vi "HandleObservationSync_002.vi"(8 "error in (no error)":errorcluster, 11 "S4GUI in":refnum<class "S4GUI.lvclass">) -> (0 "error out":errorcluster, 3 "S4GUI out":refnum<class "S4GUI.lvclass">)   [LabVIEW 2018, in "S4GUI.lvclass"] (continued)
            tunnel: ["" ("Error Msg") "ERROR: Lost channel 1 connection... - HandleObservationSync.vi state 308" ("Error Msg") "ERROR: Lost channel 2 connection...- HandleObservationSync.vi state 308" ("Error Msg") "ERROR: Lost channels 1 and 2 connection...- HandleObservationSync.vi state 308" ("Error Msg") "ERROR: Lost channel 3 connection...- HandleObservationSync.vi state 308" ("Error Msg") "ERROR: Lost channels 1 and  3 connection...- HandleObservationSync.vi state 308" ("Error Msg") "ERROR:  Lost channels 2 and  3 connection...- HandleObservationSync.vi state 308" ("Error Msg") "ERROR:  Lost channels 1, 2 and  3 connection...- HandleObservationSync.vi state 308" ("Error Msg") "ERROR: Lost channel 4 connection...- HandleObservationSync.vi state 308" ("Error Msg") "ERROR:  Lost channels 1 and 4 connection...- HandleObservationSync.vi state 308" ("Error Msg") "ERROR:  Lost channels 2 and 4 connection...- HandleObservationSync.vi state 308" ("Error Msg") "ERROR: Lost channels 1, 2 and 4 connection...- HandleObservationSync.vi state 308" ("Error Msg") "ERROR: Lost channels 3 and 4 connection...- HandleObservationSync.vi state 308" ("Error Msg") "ERROR: Lost channels 1, 3 and 4 connection...- HandleObservationSync.vi state 308" ("Error Msg") "ERROR: Lost channels 2, 3 and 4 connection...- HandleObservationSync.vi state 308" ("Error Msg") "ERROR: Lost channels 1, 2, 3 and 4 connection...- HandleObservationSync.vi state 308" ("Error Msg")] -> w2599
            frame 0, Default {
              n1014 = Tick Count (ms)() -> (millisecond timer value=w2631:u32)
              n1015 = Increment(x=w2634) -> (x+1=w2633:u32)
              n1016 = local write "time1"(w2631) -> ()
            }
            frame 1 {
            }
            frame 2 {
            }
            frame 3 {
            }
            frame 4 {
            }
            frame 5 {
            }
            frame 6 {
            }
            frame 7 {
            }
            frame 8 {
            }
            frame 9 {
            }
            frame 10 {
            }
            frame 11 {
            }
            frame 12 {
            }
            frame 13 {
            }
            frame 14 {
            }
            frame 15 {
            }
          }
          n1017 = Bundle By Name(cluster=w2608, "Obs_state"=w2598, "Error Msg"=w2599) -> (w2625:refnum<class "S4GUI.lvclass">)
        }
        frame 309 {
          # "Se wait_expose=T, não envia\no EXPOSE do estado 310\n(1o EXPOSE já foi enviado).\n\nNeste caso, vai para:\n* 310 se houver mais \n   de 1 posição da lamina ou para \n* 327 se houver apenas 1 posição\n   da lâmina"
          # "T: mode EXPOSE\nF: mode FIRE"
          # "Espera todos os canais chegarem ao estado ACTIVE\n(estados 54 e 55 de Channel:Run.vi)\n   OU\nTodos os canais incrementarem o Seqs_done. (OV 20240821)"
          n1018 = Unbundle By Name(w2754) -> ("seqAtual"=w2753:u32)
          n1019 = call-dynamic "Read AcquisitionA.vi"("error in (no error)"=w2816, "S4ACS_GUI in"=w2754) -> ("error out"=w2796:errorcluster, "Acquisition.lvclass"=w2797:refnum<class "Acquisition.lvclass">, "S4ACS_GUI out"=w2818:refnum<class "S4GUI.lvclass">)  [unwired: 7 in]
          n1020 = call "Read connection.vi"("error in (no error)"=w2796, "Server in"=w2797) -> ("error out"=w2798:errorcluster, "connection"=w2800:bool, "Server out"=w2799:refnum<class "Acquisition.lvclass">)  [unwired: 7 in]
          n1021 = case shown="True" w2800 {
            tunnel: [w2953 w2977] -> w2819
            tunnel: [w2952 w2976] -> w2817
            tunnel: w2799 -> [w2953 w2969]
            tunnel: w2798 -> [w2952 w2968]
            tunnel: [TRUE w2967] -> w2779
            tunnel: [FALSE w2961] -> w2775
            tunnel: [TRUE w2955] -> w2758
            tunnel: w2753 -> [_ w2954]
            frame False {
            }
            frame True {
              n1022 = call-dynamic "Read Channel.vi"("error in (no error)"=w2968, "Acquisition in"=w2969) -> ("error out"=w2958:errorcluster, "Channel.lvclass"=w2960:refnum<class "Channel.lvclass">, "Acquisition out"=w2978:refnum<class "Acquisition.lvclass">)  [unwired: 7 in]
              n1023 = call-dynamic "Read SequesDone.vi"("error in (no error)"=w2958, "Channel in"=w2960) -> ("error out"=w2957:errorcluster, "SequesDoneRaw"=w2956:u32, "Channel out"=w2959:refnum<class "Channel.lvclass">)  [unwired: 6 in, 1 out]
              n1024 = Equal?(x=w2956, y=w2954) -> (x = y?=w2955:bool)
              n1025 = call-dynamic "Read wait_expose.vi"("error in (no error)"=w2957, "Channel in"=w2959) -> ("error out"=w2962:errorcluster, "wait_expose"=w2961:bool, "Channel out"=w2963:refnum<class "Channel.lvclass">)  [unwired: 7 in]
              n1026 = call-dynamic "Read State Machine.vi"("error in (no error)"=w2962, "Device in"=w2963) -> ("error out"=w2970:errorcluster, "State Machine.lvclass"=w2972:refnum<class "State Machine.lvclass">, "Device out"=w2974:refnum<class "Channel.lvclass">)  [unwired: 7 in]
              n1027 = call-dynamic "Read State.vi"("error in (no error)"=w2970, "State Machine in"=w2972) -> ("error out"=w2964:errorcluster, "State"=w2966:i32, "State Machine out"=w2971:refnum<class "State Machine.lvclass">)  [unwired: 7 in]
              n1028 = Greater?(x=w2966, y=53) -> (0:w2967:bool)
              n1029 = call-dynamic "Write State Machine.vi"("error in (no error)"=w2964, "State Machine.lvclass"=w2971, "Device in"=w2974) -> ("error out"=w2973:errorcluster, "Device out"=w2975:refnum<class "Channel.lvclass">)  [unwired: 7 in]
              n1030 = call-dynamic "Write Channel.vi"("error in (no error)"=w2973, "Channel.lvclass"=w2975, "Acquisition in"=w2978) -> ("error out"=w2976:errorcluster, "Acquisition out"=w2977:refnum<class "Acquisition.lvclass">)  [unwired: 7 in]
            }
          }
          n1031 = call-dynamic "Write AcquisitionA.vi"("error in (no error)"=w2817, "Acquisition.lvclass"=w2819, "S4ACS_GUI in"=w2818) -> ("error out"=w2813:errorcluster, "S4ACS_GUI out"=w2814:refnum<class "S4GUI.lvclass">)  [unwired: 7 in]
          n1032 = call "Read AcquisitionB.vi"("error in (no error)"=w2813, "S4ACS_GUI in"=w2814) -> ("error out"=w2793:errorcluster, "Acquisition.lvclass"=w2795:refnum<class "Acquisition.lvclass">, "S4ACS_GUI out"=w2811:refnum<class "S4GUI.lvclass">)  [unwired: 7 in]
          n1033 = call "Read connection.vi"("error in (no error)"=w2793, "Server in"=w2795) -> ("error out"=w2792:errorcluster, "connection"=w2791:bool, "Server out"=w2794:refnum<class "Acquisition.lvclass">)  [unwired: 7 in]
          n1034 = case shown="True" w2791 {
            tunnel: w2794 -> [w2923 w2948]
            tunnel: w2792 -> [w2922 w2947]
            tunnel: [w2923 w2945] -> w2812
            tunnel: [w2922 w2944] -> w2810
            tunnel: [TRUE w2935] -> w2778
            tunnel: [FALSE ("expose") w2931] -> w2774
            tunnel: [TRUE w2925] -> w2760
            tunnel: w2753 -> [_ w2924]
            frame False {
            }
            frame True {
              n1035 = call-dynamic "Read Channel.vi"("error in (no error)"=w2947, "Acquisition in"=w2948) -> ("error out"=w2927:errorcluster, "Channel.lvclass"=w2930:refnum<class "Channel.lvclass">, "Acquisition out"=w2946:refnum<class "Acquisition.lvclass">)  [unwired: 7 in]
              n1036 = call-dynamic "Read SequesDone.vi"("error in (no error)"=w2927, "Channel in"=w2930) -> ("error out"=w2926:errorcluster, "SequesDoneRaw"=w2928:u32, "Channel out"=w2929:refnum<class "Channel.lvclass">)  [unwired: 6 in, 1 out]
              n1037 = Equal?(x=w2928, y=w2924) -> (x = y?=w2925:bool)
              n1038 = call-dynamic "Read wait_expose.vi"("error in (no error)"=w2926, "Channel in"=w2929) -> ("error out"=w2932:errorcluster, "wait_expose"=w2931:bool, "Channel out"=w2933:refnum<class "Channel.lvclass">)  [unwired: 7 in]
              n1039 = call-dynamic "Read State Machine.vi"("error in (no error)"=w2932, "Device in"=w2933) -> ("error out"=w2938:errorcluster, "State Machine.lvclass"=w2940:refnum<class "State Machine.lvclass">, "Device out"=w2942:refnum<class "Channel.lvclass">)  [unwired: 7 in]
              n1040 = call-dynamic "Read State.vi"("error in (no error)"=w2938, "State Machine in"=w2940) -> ("error out"=w2937:errorcluster, "State"=w2934:i32, "State Machine out"=w2939:refnum<class "State Machine.lvclass">)  [unwired: 7 in]
              n1041 = Greater?(x=w2934, y=53) -> (0:w2935:bool)
              n1042 = call-dynamic "Write State Machine.vi"("error in (no error)"=w2937, "State Machine.lvclass"=w2939, "Device in"=w2942) -> ("error out"=w2941:errorcluster, "Device out"=w2943:refnum<class "Channel.lvclass">)  [unwired: 7 in]
              n1043 = call-dynamic "Write Channel.vi"("error in (no error)"=w2941, "Channel.lvclass"=w2943, "Acquisition in"=w2946) -> ("error out"=w2944:errorcluster, "Acquisition out"=w2945:refnum<class "Acquisition.lvclass">)  [unwired: 7 in]
            }
          }
          n1044 = call "Write AcquisitionB.vi"("error in (no error)"=w2810, "Acquisition.lvclass"=w2812, "S4ACS_GUI in"=w2811) -> ("error out"=w2806:errorcluster, "S4ACS_GUI out"=w2805:refnum<class "S4GUI.lvclass">)  [unwired: 7 in]
          n1045 = call-dynamic "Read AcquisitionC.vi"("error in (no error)"=w2806, "S4ACS_GUI in"=w2805) -> ("error out"=w2788:errorcluster, "Acquisition.lvclass"=w2790:refnum<class "Acquisition.lvclass">, "S4ACS_GUI out"=w2808:refnum<class "S4GUI.lvclass">)  [unwired: 7 in]
          n1046 = call "Read connection.vi"("error in (no error)"=w2788, "Server in"=w2790) -> ("error out"=w2787:errorcluster, "connection"=w2786:bool, "Server out"=w2789:refnum<class "Acquisition.lvclass">)  [unwired: 7 in]
          n1047 = case shown="True" w2786 {
            tunnel: [w2892 w2913] -> w2809
            tunnel: [w2893 w2912] -> w2807
            tunnel: w2789 -> [w2893 w2908]
            tunnel: w2787 -> [w2892 w2907]
            tunnel: [TRUE w2904] -> w2777
            tunnel: [FALSE ("expose") w2901] -> w2773
            tunnel: [TRUE w2895] -> w2759
            tunnel: w2753 -> [_ w2894]
            frame False {
            }
            frame True {
              n1048 = call-dynamic "Read Channel.vi"("error in (no error)"=w2907, "Acquisition in"=w2908) -> ("error out"=w2900:errorcluster, "Channel.lvclass"=w2899:refnum<class "Channel.lvclass">, "Acquisition out"=w2911:refnum<class "Acquisition.lvclass">)  [unwired: 7 in]
              n1049 = call-dynamic "Read SequesDone.vi"("error in (no error)"=w2900, "Channel in"=w2899) -> ("error out"=w2896:errorcluster, "SequesDoneRaw"=w2897:u32, "Channel out"=w2898:refnum<class "Channel.lvclass">)  [unwired: 6 in, 1 out]
              n1050 = Equal?(x=w2897, y=w2894) -> (x = y?=w2895:bool)
              n1051 = call-dynamic "Read wait_expose.vi"("error in (no error)"=w2896, "Channel in"=w2898) -> ("error out"=w2902:errorcluster, "wait_expose"=w2901:bool, "Channel out"=w2903:refnum<class "Channel.lvclass">)  [unwired: 7 in]
              n1052 = call-dynamic "Read State Machine.vi"("error in (no error)"=w2902, "Device in"=w2903) -> ("error out"=w2909:errorcluster, "State Machine.lvclass"=w2917:refnum<class "State Machine.lvclass">, "Device out"=w2915:refnum<class "Channel.lvclass">)  [unwired: 7 in]
              n1053 = call-dynamic "Read State.vi"("error in (no error)"=w2909, "State Machine in"=w2917) -> ("error out"=w2910:errorcluster, "State"=w2905:i32, "State Machine out"=w2918:refnum<class "State Machine.lvclass">)  [unwired: 7 in]
              n1054 = Greater?(x=w2905, y=53) -> (0:w2904:bool)
              n1055 = call-dynamic "Write State Machine.vi"("error in (no error)"=w2910, "State Machine.lvclass"=w2918, "Device in"=w2915) -> ("error out"=w2916:errorcluster, "Device out"=w2914:refnum<class "Channel.lvclass">)  [unwired: 7 in]
              n1056 = call-dynamic "Write Channel.vi"("error in (no error)"=w2916, "Channel.lvclass"=w2914, "Acquisition in"=w2911) -> ("error out"=w2913:errorcluster, "Acquisition out"=w2912:refnum<class "Acquisition.lvclass">)  [unwired: 7 in]
            }
          }
          n1057 = call-dynamic "Write AcquisitionC.vi"("error in (no error)"=w2809, "Acquisition.lvclass"=w2807, "S4ACS_GUI in"=w2808) -> ("error out"=w2785:errorcluster, "S4ACS_GUI out"=w2801:refnum<class "S4GUI.lvclass">)  [unwired: 7 in]
          n1058 = call-dynamic "Read AcquisitionD.vi"("error in (no error)"=w2785, "S4ACS_GUI in"=w2801) -> ("error out"=w2781:errorcluster, "Acquisition.lvclass"=w2784:refnum<class "Acquisition.lvclass">, "S4ACS_GUI out"=w2803:refnum<class "S4GUI.lvclass">)  [unwired: 7 in]
          n1059 = call "Read connection.vi"("error in (no error)"=w2781, "Server in"=w2784) -> ("error out"=w2782:errorcluster, "connection"=w2780:bool, "Server out"=w2783:refnum<class "Acquisition.lvclass">)  [unwired: 7 in]
          n1060 = case shown="True" w2780 {
            tunnel: [w2863 w2887] -> w2804
            tunnel: [w2862 w2886] -> w2802
            tunnel: [TRUE w2875] -> w2776
            tunnel: w2783 -> [w2863 w2878]
            tunnel: w2782 -> [w2862 w2877]
            tunnel: [FALSE ("expose") w2871] -> w2772
            tunnel: [TRUE w2865] -> w2761
            tunnel: w2753 -> [_ w2864]
            frame False {
            }
            frame True {
              n1061 = call-dynamic "Read Channel.vi"("error in (no error)"=w2877, "Acquisition in"=w2878) -> ("error out"=w2869:errorcluster, "Channel.lvclass"=w2870:refnum<class "Channel.lvclass">, "Acquisition out"=w2888:refnum<class "Acquisition.lvclass">)  [unwired: 7 in]
              n1062 = call-dynamic "Read SequesDone.vi"("error in (no error)"=w2869, "Channel in"=w2870) -> ("error out"=w2867:errorcluster, "SequesDoneRaw"=w2868:u32, "Channel out"=w2866:refnum<class "Channel.lvclass">)  [unwired: 6 in, 1 out]
              n1063 = Equal?(x=w2868, y=w2864) -> (x = y?=w2865:bool)
              n1064 = call-dynamic "Read wait_expose.vi"("error in (no error)"=w2867, "Channel in"=w2866) -> ("error out"=w2872:errorcluster, "wait_expose"=w2871:bool, "Channel out"=w2873:refnum<class "Channel.lvclass">)  [unwired: 7 in]
              n1065 = call-dynamic "Read State Machine.vi"("error in (no error)"=w2872, "Device in"=w2873) -> ("error out"=w2880:errorcluster, "State Machine.lvclass"=w2882:refnum<class "State Machine.lvclass">, "Device out"=w2884:refnum<class "Channel.lvclass">)  [unwired: 7 in]
              n1066 = call-dynamic "Read State.vi"("error in (no error)"=w2880, "State Machine in"=w2882) -> ("error out"=w2879:errorcluster, "State"=w2874:i32, "State Machine out"=w2881:refnum<class "State Machine.lvclass">)  [unwired: 7 in]
              n1067 = Greater?(x=w2874, y=53) -> (0:w2875:bool)
              n1068 = call-dynamic "Write State Machine.vi"("error in (no error)"=w2879, "State Machine.lvclass"=w2881, "Device in"=w2884) -> ("error out"=w2883:errorcluster, "Device out"=w2885:refnum<class "Channel.lvclass">)  [unwired: 7 in]
              n1069 = call-dynamic "Write Channel.vi"("error in (no error)"=w2883, "Channel.lvclass"=w2885, "Acquisition in"=w2888) -> ("error out"=w2886:errorcluster, "Acquisition out"=w2887:refnum<class "Acquisition.lvclass">)  [unwired: 7 in]
            }
          }
          n1070 = call-dynamic "Write AcquisitionD.vi"("error in (no error)"=w2802, "Acquisition.lvclass"=w2804, "S4ACS_GUI in"=w2803) -> ("error out"=w2770:errorcluster, "S4ACS_GUI out"=w2771:refnum<class "S4GUI.lvclass">)  [unwired: 7 in]
          n1071 = Compound Arithmetic op=OR(w2775, w2774, w2773, w2772) -> (w2763:bool)
          n1072 = Compound Arithmetic op=AND(w2758, w2760, w2759, w2761) -> (w2756:bool)
          n1073 = Compound Arithmetic op=AND(w2779, w2778, w2777, w2776) -> (w2757:bool)
          n1074 = Or(x=w2757, y=w2756) -> (x .or. y?=w2755:bool)
          n1075 = call-dynamic "VerifWavePlate.vi"("error in (no error)"=w2770, "S4GUI in"=w2771) -> ("error out"=w2767:errorcluster, "One Position"=w2769:bool, "S4GUI out"=w2768:refnum<class "S4GUI.lvclass">)  [unwired: 7 in]
          n1076 = case shown="True" w2769 {
            tunnel: w2768 -> [w2840 w2857]
            tunnel: [u32 312 ("t") u32 327 ("t")] -> w2765
            tunnel: [w2840 w2843] -> w2764
            tunnel: w2767 -> [w2838 w2842]
            tunnel: [w2838 w2841] -> w2766
            frame False {
            }
            frame True {
              # "Recarrega SEQ, antes de desviar\n para tratamento de fotometria."
              n1077 = call "Read Instrument.lvclass.vi"("error in (no error)"=w2842, "S4ACS_GUI in"=w2857) -> ("error out"=w2852:errorcluster, "Instrument.lvclass"=w2856:refnum<class "Instrument.lvclass">, "S4ACS_GUI out"=w2855:refnum<class "S4GUI.lvclass">)  [unwired: 7 in]
              n1078 = call "Read WPROT.vi"("error in (no error)"=w2852, "Instrument in"=w2856) -> ("error out"=w2845:errorcluster, "Opt_Selector.lvclass"=w2848:refnum<class "Opt_Selector.lvclass">, "Instrument out"=w2853:refnum<class "Instrument.lvclass">)  [unwired: 7 in]
              n1079 = call-dynamic "Read sequencia_ant.vi"("error in (no error)"=w2845, "Opt_Selector in"=w2848) -> ("error out"=w2850:errorcluster, "sequencia_ant"=w2849:u16, "Opt_Selector out"=w2847:refnum<class "Opt_Selector.lvclass">)  [unwired: 7 in]
              n1080 = call-dynamic "Write sequencia.vi"("error in (no error)"=w2850, "sequencia"=w2849, "Opt_Selector in"=w2847) -> ("error out"=w2844:errorcluster, "Opt_Selector out"=w2846:refnum<class "Opt_Selector.lvclass">)  [unwired: 7 in]
              n1081 = call "Write WPROT.vi"("error in (no error)"=w2844, "Opt_Selector.lvclass"=w2846, "Instrument in"=w2853) -> ("error out"=w2851:errorcluster, "Instrument out"=w2854:refnum<class "Instrument.lvclass">)  [unwired: 7 in]
              n1082 = call "Write Instrument.lvclass.vi"("error in (no error)"=w2851, "Instrument.lvclass"=w2854, "S4ACS_GUI in"=w2855) -> ("error out"=w2841:errorcluster, "S4ACS_GUI out"=w2843:refnum<class "S4GUI.lvclass">)  [unwired: 7 in]
            }
          }
          n1083 = case shown="True" w2755 {
            tunnel: w2764 -> [w2821 w2837]
            tunnel: [w2827 w2836] -> w2762
            tunnel: w2765 -> [_ w2834]
            frame False {
              # "Aguardando iniciar exposição por 5s"
              n1084 = Tick Count (ms)() -> (millisecond timer value=w2826:u32)
              n1085 = local read "time1"() -> (w2820:u32)
              n1086 = Subtract(x=w2826, y=w2820) -> (x-y=w2823:u32)
              n1087 = To Double Precision Float(number=w2823) -> (double precision float=w2825:dbl)
              n1088 = Less?(x=5000.0 ("y"), y=w2825) -> (x < y?=w2824:bool)
              n1089 = case shown="True" w2824 {
                tunnel: w2821 -> [w2828 w2832]
                tunnel: [w2828 w2831] -> w2827
                frame False {
                }
                frame True {
                  n1090 = Bundle By Name(cluster=w2832, "Obs_state"=u32 1, "Error Msg"="ERROR: Acquisition Timeout. HandleObservationSync.vi - state 309.") -> (w2831:refnum<class "S4GUI.lvclass">)
                }
              }
            }
            frame True {
              # "Iniciou aquisição..."
              n1091 = Tick Count (ms)() -> (millisecond timer value=→"time308":u32)
              n1092 = Tick Count (ms)() -> (millisecond timer value=w2835:u32)
              n1093 = Bundle By Name(cluster=w2837, "Obs_state"=w2834) -> (w2836:refnum<class "S4GUI.lvclass">)
              n1094 = local write "time307"(w2835) -> ()
              n1095 = local write "time1"(w2835) -> ()
            }
          }
          n1096 = Bundle By Name(cluster=w2762, "mode EXPOSE"=w2763) -> (w2815:refnum<class "S4GUI.lvclass">)
        }
        frame 312 {
          # "Verifcando avanço de SEQUENCIA:"
          # "T=canais receberam STOP"
          # "T= Todos os canais ativos na mesma sequencia;\nF= Canais com sequencia diferente"
          # "Todos os SEQ_DONE \nsão iguais a SeqAtual?\nSe sim, avança lâmina."
          # "Exemplo:\nSET #CYCLES 3\nSET #SEQ 4\ntotal de sequencias: 3 x 4 = 12\n\nseq.        CYCLES_DONE           SEQS_DONE\n1a.                     0                                 0\n2a.                     0                                 1 \n3a.                     0                                 2 \n4a.                     0                                 3 \n                          1                                 4\n5a.                     1                                 0 \n6a.                     1                                 1 \n7a.                     1                                 2 \n8a.                     1                                 3 \n                          2                                 4\n9a.                     2                                 0 \n10a.                   2                                 1 \n11a.                   2                                 2 \n12a.                   2                                 3 \n\nfim                    3                                 4"
          n1097 = Unbundle By Name(w3004) -> ("seqAtual"=w3001:u32)
          n1098 = call-dynamic "Read AcquisitionA.vi"("error in (no error)"=w3038, "S4ACS_GUI in"=w3004) -> ("error out"=w3019:errorcluster, "Acquisition.lvclass"=w3020:refnum<class "Acquisition.lvclass">, "S4ACS_GUI out"=w3040:refnum<class "S4GUI.lvclass">)  [unwired: 7 in]
          n1099 = call-dynamic "Read enabled.vi"("error in (no error)"=w3019, "Server in"=w3020) -> ("error out"=w3018:errorcluster, "enabled"=w2993:bool, "Server out"=w3017:refnum<class "Acquisition.lvclass">)  [unwired: 7 in]
          n1100 = case shown="True" w2993 {
            tunnel: w3018 -> [w3189 w3205]
            tunnel: [w3190 w3203] -> w3041
            tunnel: [w3189 w3202] -> w3039
            tunnel: [u32 0 ("SequesDone") w3191] -> w2998
            tunnel: w3017 -> [w3190 w3201]
            tunnel: w3001 -> [_ w3200]
            tunnel: [TRUE w3199] -> w3003
            tunnel: [FALSE ("stopping") w3192] -> w2986
            frame False {
            }
            frame True {
              # "SEQS_DONE = 0,1,2,...,n,0,1,..."
              n1101 = call-dynamic "Read Channel.vi"("error in (no error)"=w3205, "Acquisition in"=w3201) -> ("error out"=w3197:errorcluster, "Channel.lvclass"=w3198:refnum<class "Channel.lvclass">, "Acquisition out"=w3204:refnum<class "Acquisition.lvclass">)  [unwired: 7 in]
              n1102 = call-dynamic "Read SequesDone.vi"("error in (no error)"=w3197, "Channel in"=w3198) -> ("error out"=w3195:errorcluster, "SequesDoneRaw"=w3191:u32, "Channel out"=w3196:refnum<class "Channel.lvclass">)  [unwired: 6 in, 1 out]
              n1103 = Equal?(x=w3191, y=w3200) -> (x = y?=w3199:bool)
              n1104 = call-dynamic "Read stopping.vi"("error in (no error)"=w3195, "Channel in"=w3196) -> ("error out"=w3194:errorcluster, "stopping"=w3192:bool, "Channel out"=w3193:refnum<class "Channel.lvclass">)  [unwired: 7 in]
              n1105 = call-dynamic "Write Channel.vi"("error in (no error)"=w3194, "Channel.lvclass"=w3193, "Acquisition in"=w3204) -> ("error out"=w3202:errorcluster, "Acquisition out"=w3203:refnum<class "Acquisition.lvclass">)  [unwired: 7 in]
            }
          }
          n1106 = call-dynamic "Write AcquisitionA.vi"("error in (no error)"=w3039, "Acquisition.lvclass"=w3041, "S4ACS_GUI in"=w3040) -> ("error out"=w3036:errorcluster, "S4ACS_GUI out"=w3035:refnum<class "S4GUI.lvclass">)  [unwired: 7 in]
          n1107 = call "Read AcquisitionB.vi"("error in (no error)"=w3036, "S4ACS_GUI in"=w3035) -> ("error out"=w3013:errorcluster, "Acquisition.lvclass"=w3016:refnum<class "Acquisition.lvclass">, "S4ACS_GUI out"=w3037:refnum<class "S4GUI.lvclass">)  [unwired: 7 in]
          n1108 = call-dynamic "Read enabled.vi"("error in (no error)"=w3013, "Server in"=w3016) -> ("error out"=w3014:errorcluster, "enabled"=w2992:bool, "Server out"=w3015:refnum<class "Acquisition.lvclass">)  [unwired: 7 in]
          n1109 = case shown="True" w2992 {
            tunnel: w3014 -> [w3169 w3185]
            tunnel: w3015 -> [w3170 w3184]
            tunnel: [u32 0 ("SequesDone") w3171] -> w2995
            tunnel: [w3169 w3183] -> w3034
            tunnel: [w3170 w3182] -> w3033
            tunnel: w3001 -> [_ w3179]
            tunnel: [TRUE w3178] -> w3002
            tunnel: [FALSE ("stopping") w3172] -> w2985
            frame False {
            }
            frame True {
              n1110 = call-dynamic "Read Channel.vi"("error in (no error)"=w3185, "Acquisition in"=w3184) -> ("error out"=w3176:errorcluster, "Channel.lvclass"=w3177:refnum<class "Channel.lvclass">, "Acquisition out"=w3180:refnum<class "Acquisition.lvclass">)  [unwired: 7 in]
              n1111 = call-dynamic "Read SequesDone.vi"("error in (no error)"=w3176, "Channel in"=w3177) -> ("error out"=w3174:errorcluster, "SequesDoneRaw"=w3171:u32, "Channel out"=w3181:refnum<class "Channel.lvclass">)  [unwired: 6 in, 1 out]
              n1112 = Equal?(x=w3171, y=w3179) -> (x = y?=w3178:bool)
              n1113 = call-dynamic "Read stopping.vi"("error in (no error)"=w3174, "Channel in"=w3181) -> ("error out"=w3173:errorcluster, "stopping"=w3172:bool, "Channel out"=w3175:refnum<class "Channel.lvclass">)  [unwired: 7 in]
              n1114 = call-dynamic "Write Channel.vi"("error in (no error)"=w3173, "Channel.lvclass"=w3175, "Acquisition in"=w3180) -> ("error out"=w3183:errorcluster, "Acquisition out"=w3182:refnum<class "Acquisition.lvclass">)  [unwired: 7 in]
            }
          }
          n1115 = call "Write AcquisitionB.vi"("error in (no error)"=w3034, "Acquisition.lvclass"=w3033, "S4ACS_GUI in"=w3037) -> ("error out"=w3026:errorcluster, "S4ACS_GUI out"=w3025:refnum<class "S4GUI.lvclass">)  [unwired: 7 in]
          n1116 = call-dynamic "Read AcquisitionC.vi"("error in (no error)"=w3026, "S4ACS_GUI in"=w3025) -> ("error out"=w3010:errorcluster, "Acquisition.lvclass"=w3012:refnum<class "Acquisition.lvclass">, "S4ACS_GUI out"=w3028:refnum<class "S4GUI.lvclass">)  [unwired: 7 in]
          n1117 = call-dynamic "Read enabled.vi"("error in (no error)"=w3010, "Server in"=w3012) -> ("error out"=w3009:errorcluster, "enabled"=w2991:bool, "Server out"=w3011:refnum<class "Acquisition.lvclass">)  [unwired: 7 in]
          n1118 = case shown="True" w2991 {
            tunnel: [w3149 w3165] -> w3029
            tunnel: [w3150 w3164] -> w3027
            tunnel: w3009 -> [w3149 w3161]
            tunnel: w3011 -> [w3150 w3162]
            tunnel: [u32 0 ("SequesDone") w3151] -> w2994
            tunnel: w3001 -> [_ w3160]
            tunnel: [TRUE w3159] -> w3000
            tunnel: [FALSE ("stopping") w3152] -> w2984
            frame False {
            }
            frame True {
              n1119 = call-dynamic "Read Channel.vi"("error in (no error)"=w3161, "Acquisition in"=w3162) -> ("error out"=w3156:errorcluster, "Channel.lvclass"=w3157:refnum<class "Channel.lvclass">, "Acquisition out"=w3163:refnum<class "Acquisition.lvclass">)  [unwired: 7 in]
              n1120 = call-dynamic "Read SequesDone.vi"("error in (no error)"=w3156, "Channel in"=w3157) -> ("error out"=w3154:errorcluster, "SequesDoneRaw"=w3151:u32, "Channel out"=w3158:refnum<class "Channel.lvclass">)  [unwired: 6 in, 1 out]
              n1121 = Equal?(x=w3151, y=w3160) -> (x = y?=w3159:bool)
              n1122 = call-dynamic "Read stopping.vi"("error in (no error)"=w3154, "Channel in"=w3158) -> ("error out"=w3153:errorcluster, "stopping"=w3152:bool, "Channel out"=w3155:refnum<class "Channel.lvclass">)  [unwired: 7 in]
              n1123 = call-dynamic "Write Channel.vi"("error in (no error)"=w3153, "Channel.lvclass"=w3155, "Acquisition in"=w3163) -> ("error out"=w3165:errorcluster, "Acquisition out"=w3164:refnum<class "Acquisition.lvclass">)  [unwired: 7 in]
            }
          }
          n1124 = call-dynamic "Write AcquisitionC.vi"("error in (no error)"=w3029, "Acquisition.lvclass"=w3027, "S4ACS_GUI in"=w3028) -> ("error out"=w3023:errorcluster, "S4ACS_GUI out"=w3024:refnum<class "S4GUI.lvclass">)  [unwired: 7 in]
          n1125 = call-dynamic "Read AcquisitionD.vi"("error in (no error)"=w3023, "S4ACS_GUI in"=w3024) -> ("error out"=w3006:errorcluster, "Acquisition.lvclass"=w3008:refnum<class "Acquisition.lvclass">, "S4ACS_GUI out"=w3030:refnum<class "S4GUI.lvclass">)  [unwired: 7 in]
          n1126 = call-dynamic "Read enabled.vi"("error in (no error)"=w3006, "Server in"=w3008) -> ("error out"=w3005:errorcluster, "enabled"=w2990:bool, "Server out"=w3007:refnum<class "Acquisition.lvclass">)  [unwired: 7 in]
          n1127 = Build Array(w2993, w2992, w2991, w2990) -> (w2989:bool[])
          n1128 = case shown="True" w2990 {
            tunnel: [w3130 w3145] -> w3032
            tunnel: [w3129 w3144] -> w3031
            tunnel: w3007 -> [w3130 w3143]
            tunnel: w3005 -> [w3129 w3142]
            tunnel: [u32 0 ("SequesDone") w3131] -> w2997
            tunnel: w3001 -> [_ w3140]
            tunnel: [TRUE w3139] -> w2999
            tunnel: [FALSE ("stopping") w3132] -> w2983
            frame False {
            }
            frame True {
              n1129 = call-dynamic "Read Channel.vi"("error in (no error)"=w3142, "Acquisition in"=w3143) -> ("error out"=w3136:errorcluster, "Channel.lvclass"=w3137:refnum<class "Channel.lvclass">, "Acquisition out"=w3141:refnum<class "Acquisition.lvclass">)  [unwired: 7 in]
              n1130 = call-dynamic "Read SequesDone.vi"("error in (no error)"=w3136, "Channel in"=w3137) -> ("error out"=w3134:errorcluster, "SequesDoneRaw"=w3131:u32, "Channel out"=w3138:refnum<class "Channel.lvclass">)  [unwired: 6 in, 1 out]
              n1131 = Equal?(x=w3131, y=w3140) -> (x = y?=w3139:bool)
              n1132 = call-dynamic "Read stopping.vi"("error in (no error)"=w3134, "Channel in"=w3138) -> ("error out"=w3133:errorcluster, "stopping"=w3132:bool, "Channel out"=w3135:refnum<class "Channel.lvclass">)  [unwired: 7 in]
              n1133 = call-dynamic "Write Channel.vi"("error in (no error)"=w3133, "Channel.lvclass"=w3135, "Acquisition in"=w3141) -> ("error out"=w3144:errorcluster, "Acquisition out"=w3145:refnum<class "Acquisition.lvclass">)  [unwired: 7 in]
            }
          }
          n1134 = Boolean Array To Number(Boolean array=w2989) -> (number=w2987:u32)
          n1135 = Compound Arithmetic op=AND(w3003, w3002, w3000, w2999) -> (w2988:bool)
          n1136 = Compound Arithmetic op=OR(w2986, w2985, w2984, w2983) -> (w2982:bool)
          n1137 = case shown="11" w2987 {
            tunnel: w2998 -> [w3049 _ w3061 _ w3070 _ w3076 w3082 _ w3088 w3091 _]
            tunnel: w2997 -> [w3048 w3052 w3057 w3064 w3065 w3073 w3075 _ _ _ _ _]
            tunnel: w2995 -> [w3047 w3050 _ _ w3069 w3071 _ w3081 w3085 _ w3090 _]
            tunnel: w2994 -> [w3046 w3051 w3056 w3062 _ _ _ w3080 w3084 w3087 _ _]
            tunnel: [w3042 w3053 w3058 w3063 w3066 w3072 w3074 w3077 w3083 w3086 w3089 TRUE] -> _
            frame 15 {
              # "A,B,C,D ativos"
              n1138 = Equal?(x=w3049, y=w3047) -> (x = y?=w3045:bool)
              n1139 = Equal?(x=w3046, y=w3048) -> (x = y?=w3043:bool)
              n1140 = Equal?(x=w3047, y=w3046) -> (x = y?=w3044:bool)
              n1141 = Compound Arithmetic op=AND(w3045, w3044, w3043) -> (w3042:bool)
            }
            frame 14 {
              # "B,C e,D ativos"
              n1142 = Equal?(x=w3050, y=w3051) -> (x = y?=w3055:bool)
              n1143 = Equal?(x=w3051, y=w3052) -> (x = y?=w3054:bool)
              n1144 = Compound Arithmetic op=AND(w3055, w3054) -> (w3053:bool)
            }
            frame 13 {
              # "A,C e,D ativos"
              n1145 = Equal?(x=w3061, y=w3056) -> (x = y?=w3060:bool)
              n1146 = Equal?(x=w3056, y=w3057) -> (x = y?=w3059:bool)
              n1147 = Compound Arithmetic op=AND(w3060, w3059) -> (w3058:bool)
            }
            frame 12 {
              # "Só C e D ativos"
              n1148 = Equal?(x=w3062, y=w3064) -> (x = y?=w3063:bool)
            }
            frame 11 {
              # "A,B e,D ativos"
              n1149 = Equal?(x=w3070, y=w3069) -> (x = y?=w3068:bool)
              n1150 = Equal?(x=w3069, y=w3065) -> (x = y?=w3067:bool)
              n1151 = Compound Arithmetic op=AND(w3068, w3067) -> (w3066:bool)
            }
            frame 10 {
              # "Só B e D ativos"
              n1152 = Equal?(x=w3071, y=w3073) -> (x = y?=w3072:bool)
            }
            frame 9 {
              # "Só A e D ativos"
              n1153 = Equal?(x=w3076, y=w3075) -> (x = y?=w3074:bool)
            }
            frame 7 {
              # "A,B,C ativos"
              n1154 = Equal?(x=w3082, y=w3081) -> (x = y?=w3079:bool)
              n1155 = Equal?(x=w3081, y=w3080) -> (x = y?=w3078:bool)
              n1156 = Compound Arithmetic op=AND(w3079, w3078) -> (w3077:bool)
            }
            frame 6 {
              # "Só B e C ativos"
              n1157 = Equal?(x=w3085, y=w3084) -> (x = y?=w3083:bool)
            }
            frame 5 {
              # "Só A e C ativos"
              n1158 = Equal?(x=w3088, y=w3087) -> (x = y?=w3086:bool)
            }
            frame 3 {
              # "só A e B ativos"
              n1159 = Equal?(x=w3091, y=w3090) -> (x = y?=w3089:bool)
            }
            frame 0..2, 4, 8, Default {
              # "nenhum ou só 1  \ncanal ativo."
            }
          }
          n1160 = call-dynamic "Write AcquisitionD.vi"("error in (no error)"=w3031, "Acquisition.lvclass"=w3032, "S4ACS_GUI in"=w3030) -> ("error out"=w3021:errorcluster, "S4ACS_GUI out"=w3022:refnum<class "S4GUI.lvclass">)  [unwired: 7 in]
          n1161 = And(x=w2988, y=TRUE) -> (x .and. y?=w2996:bool)
          n1162 = case shown="True" w2996 {
            tunnel: w3022 -> [w3094 w3123]
            tunnel: [w3093 w3122] -> w2981
            tunnel: w2988 -> [w3095 _]
            tunnel: w2982 -> [_ w3121]
            tunnel: w2980 -> [_ w3116]
            frame False {
              n1163 = case shown="False" w3095 {
                tunnel: w3094 -> [w3102 w3115]
                tunnel: [w3106 w3114] -> w3093
                frame False {
                  # "Esperando todos os canais habilitados mudarem de sequesDone.\nE verificando a maior duracao de cubo entre os canais."
                  n1164 = local read "time307"() -> (w3105:u32)
                  n1165 = Tick Count (ms)() -> (millisecond timer value=w3104:u32)
                  n1166 = Subtract(x=w3104, y=w3105) -> (x-y=w3099:u32)
                  n1167 = call-dynamic "GetGreatestCube.vi"("S4GUI in"=w3102) -> ("S4GUI out"=w3101:refnum<class "S4GUI.lvclass">, "greatest (ms)"=w3097:dbl)  [unwired: 8 in, 1 out]
                  n1168 = To Double Precision Float(number=w3099) -> (double precision float=w3103:dbl)
                  n1169 = Add(x=1000.0 ("y"), y=w3097) -> (x+y=w3096:dbl)
                  n1170 = Less?(x=w3096, y=w3103) -> (x < y?=w3100:bool)
                  n1171 = case shown="True" w3100 {
                    tunnel: w3101 -> [w3107 w3111]
                    tunnel: [w3107 w3110] -> w3106
                    frame False {
                    }
                    frame True {
                      n1172 = Bundle By Name(cluster=w3111, "Obs_state"=u32 1, "Error Msg"="ERROR: Acquisition Timeout - HandleObservationSync.vi - state 312.") -> (w3110:refnum<class "S4GUI.lvclass">)
                    }
                  }
                }
                frame True {
                  # "Nunca entra aqui!!"
                  n1173 = Bundle By Name(cluster=w3115, "Obs_state"=u32 1, "Error Msg"="ERROR: Sequence_done not equal in all active channels.") -> (w3114:refnum<class "S4GUI.lvclass">)
                }
              }
            }
            frame True {
              # "STOP?"
              n1174 = local read "time308"() -> (w3119:u32)
              n1175 = Tick Count (ms)() -> (millisecond timer value=w3120:u32)
              n1176 = Subtract(x=w3120, y=w3119) -> (x-y=→"delay Acq":u32)
              n1177 = case shown="False" w3121 {
                tunnel: w3116 -> [_ _]
                tunnel: [u32 303 u32 0] -> w3117
                frame False {
                }
                frame True {
                }
              }
              n1178 = Bundle By Name(cluster=w3123, "Obs_state"=w3117) -> (w3122:refnum<class "S4GUI.lvclass">)
            }
          }
        }
        frame 314 {
          n1179 = Unbundle By Name(w3209) -> ("cyclesDone"=w3207:u32)
          n1180 = Increment(x=w3207) -> (x+1=w3206:u32)
          n1181 = Bundle By Name(cluster=w3209, "cyclesDone"=w3206) -> (w3208:refnum<class "S4GUI.lvclass">)
          n1182 = Unbundle By Name(w3208) -> ("TotalCiclos"=w3216:u32, "cyclesDone"=w3215:u32)
          n1183 = Subtract(x=w3216, y=w3215) -> (x-y=w3214:u32)
          n1184 = Greater Than 0?(x=w3214) -> (x > 0?=w3213:bool)
          n1185 = Select(t=u32 303, s=w3213, f=u32 0) -> (s? t:f=w3212:u32)
          n1186 = Bundle By Name(cluster=w3208, "Obs_state"=w3212) -> (w3217:refnum<class "S4GUI.lvclass">)
        }
        frame 321 {
          n1187 = call-dynamic "Read AcquisitionA.vi"("error in (no error)"=w3281, "S4ACS_GUI in"=w3282) -> ("error out"=w3236:errorcluster, "Acquisition.lvclass"=w3237:refnum<class "Acquisition.lvclass">, "S4ACS_GUI out"=w3284:refnum<class "S4GUI.lvclass">)  [unwired: 7 in]
          n1188 = call-dynamic "Read enabled.vi"("error in (no error)"=w3236, "Server in"=w3237) -> ("error out"=w3235:errorcluster, "enabled"=w3222:bool, "Server out"=w3238:refnum<class "Acquisition.lvclass">)  [unwired: 7 in]
          n1189 = call "Read connection.vi"("error in (no error)"=w3235, "Server in"=w3238) -> ("error out"=w3261:errorcluster, "connection"=w3245:bool, "Server out"=w3262:refnum<class "Acquisition.lvclass">)  [unwired: 7 in]
          n1190 = And(x=w3245, y=w3222) -> (x .and. y?=w3246:bool)
          n1191 = case shown="True" w3246 {
            tunnel: w3262 -> [w3399 w3418]
            tunnel: w3261 -> [w3398 w3417]
            tunnel: [w3399 w3415] -> w3285
            tunnel: [w3398 w3414] -> w3283
            tunnel: [w3395 u32 0 ("New_State")] -> w3251
            tunnel: w3222 -> [w3394 _]
            frame False {
              n1192 = Select(t=u32 1, s=w3394, f=u32 0) -> (s? t:f=w3395:u32)
            }
            frame True {
              n1193 = call-dynamic "Read Channel.vi"("error in (no error)"=w3417, "Acquisition in"=w3418) -> ("error out"=w3401:errorcluster, "Channel.lvclass"=w3404:refnum<class "Channel.lvclass">, "Acquisition out"=w3416:refnum<class "Acquisition.lvclass">)  [unwired: 7 in]
              n1194 = call-dynamic "Write wait_expose.vi"("error in (no error)"=w3401, "wait_expose"=TRUE, "Channel in"=w3404) -> ("error out"=w3400:errorcluster, "Channel out"=w3403:refnum<class "Channel.lvclass">)  [unwired: 7 in]
              n1195 = call-dynamic "Read State Machine.vi"("error in (no error)"=w3400, "Device in"=w3403) -> ("error out"=w3411:errorcluster, "State Machine.lvclass"=w3413:refnum<class "State Machine.lvclass">, "Device out"=w3409:refnum<class "Channel.lvclass">)  [unwired: 7 in]
              n1196 = call "Next State.vi"("error in (no error)"=w3411, "New_State"=40, "State Machine in"=w3413) -> ("error out"=w3406:errorcluster, "State Machine out"=w3407:refnum<class "State Machine.lvclass">)  [unwired: 7 in]
              n1197 = call-dynamic "Write State Machine.vi"("error in (no error)"=w3406, "State Machine.lvclass"=w3407, "Device in"=w3409) -> ("error out"=w3408:errorcluster, "Device out"=w3410:refnum<class "Channel.lvclass">)  [unwired: 7 in]
              n1198 = call-dynamic "Write Channel.vi"("error in (no error)"=w3408, "Channel.lvclass"=w3410, "Acquisition in"=w3416) -> ("error out"=w3414:errorcluster, "Acquisition out"=w3415:refnum<class "Acquisition.lvclass">)  [unwired: 7 in]
            }
          }
          n1199 = call-dynamic "Write AcquisitionA.vi"("error in (no error)"=w3283, "Acquisition.lvclass"=w3285, "S4ACS_GUI in"=w3284) -> ("error out"=w3278:errorcluster, "S4ACS_GUI out"=w3279:refnum<class "S4GUI.lvclass">)  [unwired: 7 in]
          n1200 = call "Read AcquisitionB.vi"("error in (no error)"=w3278, "S4ACS_GUI in"=w3279) -> ("error out"=w3232:errorcluster, "Acquisition.lvclass"=w3234:refnum<class "Acquisition.lvclass">, "S4ACS_GUI out"=w3276:refnum<class "S4GUI.lvclass">)  [unwired: 7 in]
          n1201 = call-dynamic "Read enabled.vi"("error in (no error)"=w3232, "Server in"=w3234) -> ("error out"=w3231:errorcluster, "enabled"=w3221:bool, "Server out"=w3233:refnum<class "Acquisition.lvclass">)  [unwired: 7 in]
          n1202 = call "Read connection.vi"("error in (no error)"=w3231, "Server in"=w3233) -> ("error out"=w3259:errorcluster, "connection"=w3243:bool, "Server out"=w3260:refnum<class "Acquisition.lvclass">)  [unwired: 7 in]
          n1203 = And(x=w3243, y=w3221) -> (x .and. y?=w3244:bool)
          n1204 = case shown="True" w3244 {
            tunnel: w3260 -> [w3374 w3393]
            tunnel: w3259 -> [w3373 w3392]
            tunnel: [w3374 w3390] -> w3277
            tunnel: [w3373 w3389] -> w3275
            tunnel: [w3370 u32 0 ("New_State")] -> w3250
            tunnel: w3221 -> [w3369 _]
            frame False {
              n1205 = Select(t=u32 2, s=w3369, f=u32 0) -> (s? t:f=w3370:u32)
            }
            frame True {
              n1206 = call-dynamic "Read Channel.vi"("error in (no error)"=w3392, "Acquisition in"=w3393) -> ("error out"=w3376:errorcluster, "Channel.lvclass"=w3378:refnum<class "Channel.lvclass">, "Acquisition out"=w3391:refnum<class "Acquisition.lvclass">)  [unwired: 7 in]
              n1207 = call-dynamic "Write wait_expose.vi"("error in (no error)"=w3376, "wait_expose"=TRUE, "Channel in"=w3378) -> ("error out"=w3375:errorcluster, "Channel out"=w3377:refnum<class "Channel.lvclass">)  [unwired: 7 in]
              n1208 = call-dynamic "Read State Machine.vi"("error in (no error)"=w3375, "Device in"=w3377) -> ("error out"=w3386:errorcluster, "State Machine.lvclass"=w3388:refnum<class "State Machine.lvclass">, "Device out"=w3384:refnum<class "Channel.lvclass">)  [unwired: 7 in]
              n1209 = call "Next State.vi"("error in (no error)"=w3386, "New_State"=40, "State Machine in"=w3388) -> ("error out"=w3381:errorcluster, "State Machine out"=w3382:refnum<class "State Machine.lvclass">)  [unwired: 7 in]
              n1210 = call-dynamic "Write State Machine.vi"("error in (no error)"=w3381, "State Machine.lvclass"=w3382, "Device in"=w3384) -> ("error out"=w3383:errorcluster, "Device out"=w3385:refnum<class "Channel.lvclass">)  [unwired: 7 in]
              n1211 = call-dynamic "Write Channel.vi"("error in (no error)"=w3383, "Channel.lvclass"=w3385, "Acquisition in"=w3391) -> ("error out"=w3389:errorcluster, "Acquisition out"=w3390:refnum<class "Acquisition.lvclass">)  [unwired: 7 in]
            }
          }
          n1212 = call "Write AcquisitionB.vi"("error in (no error)"=w3275, "Acquisition.lvclass"=w3277, "S4ACS_GUI in"=w3276) -> ("error out"=w3271:errorcluster, "S4ACS_GUI out"=w3270:refnum<class "S4GUI.lvclass">)  [unwired: 7 in]
          n1213 = call-dynamic "Read AcquisitionC.vi"("error in (no error)"=w3271, "S4ACS_GUI in"=w3270) -> ("error out"=w3228:errorcluster, "Acquisition.lvclass"=w3230:refnum<class "Acquisition.lvclass">, "S4ACS_GUI out"=w3273:refnum<class "S4GUI.lvclass">)  [unwired: 7 in]
          n1214 = call-dynamic "Read enabled.vi"("error in (no error)"=w3228, "Server in"=w3230) -> ("error out"=w3227:errorcluster, "enabled"=w3220:bool, "Server out"=w3229:refnum<class "Acquisition.lvclass">)  [unwired: 7 in]
          n1215 = call "Read connection.vi"("error in (no error)"=w3227, "Server in"=w3229) -> ("error out"=w3257:errorcluster, "connection"=w3240:bool, "Server out"=w3258:refnum<class "Acquisition.lvclass">)  [unwired: 7 in]
          n1216 = And(x=w3240, y=w3220) -> (x .and. y?=w3242:bool)
          n1217 = case shown="True" w3242 {
            tunnel: [w3348 w3362] -> w3274
            tunnel: [w3349 w3361] -> w3272
            tunnel: w3258 -> [w3349 w3359]
            tunnel: w3257 -> [w3348 w3358]
            tunnel: [w3345 u32 0 ("New_State")] -> w3249
            tunnel: w3220 -> [w3344 _]
            frame False {
              n1218 = Select(t=u32 4, s=w3344, f=u32 0) -> (s? t:f=w3345:u32)
            }
            frame True {
              n1219 = call-dynamic "Read Channel.vi"("error in (no error)"=w3358, "Acquisition in"=w3359) -> ("error out"=w3351:errorcluster, "Channel.lvclass"=w3353:refnum<class "Channel.lvclass">, "Acquisition out"=w3360:refnum<class "Acquisition.lvclass">)  [unwired: 7 in]
              n1220 = call-dynamic "Write wait_expose.vi"("error in (no error)"=w3351, "wait_expose"=TRUE, "Channel in"=w3353) -> ("error out"=w3350:errorcluster, "Channel out"=w3352:refnum<class "Channel.lvclass">)  [unwired: 7 in]
              n1221 = call-dynamic "Read State Machine.vi"("error in (no error)"=w3350, "Device in"=w3352) -> ("error out"=w3365:errorcluster, "State Machine.lvclass"=w3363:refnum<class "State Machine.lvclass">, "Device out"=w3367:refnum<class "Channel.lvclass">)  [unwired: 7 in]
              n1222 = call "Next State.vi"("error in (no error)"=w3365, "New_State"=40, "State Machine in"=w3363) -> ("error out"=w3357:errorcluster, "State Machine out"=w3356:refnum<class "State Machine.lvclass">)  [unwired: 7 in]
              n1223 = call-dynamic "Write State Machine.vi"("error in (no error)"=w3357, "State Machine.lvclass"=w3356, "Device in"=w3367) -> ("error out"=w3368:errorcluster, "Device out"=w3366:refnum<class "Channel.lvclass">)  [unwired: 7 in]
              n1224 = call-dynamic "Write Channel.vi"("error in (no error)"=w3368, "Channel.lvclass"=w3366, "Acquisition in"=w3360) -> ("error out"=w3362:errorcluster, "Acquisition out"=w3361:refnum<class "Acquisition.lvclass">)  [unwired: 7 in]
            }
          }
          n1225 = call-dynamic "Write AcquisitionC.vi"("error in (no error)"=w3274, "Acquisition.lvclass"=w3272, "S4ACS_GUI in"=w3273) -> ("error out"=w3268:errorcluster, "S4ACS_GUI out"=w3267:refnum<class "S4GUI.lvclass">)  [unwired: 7 in]
          n1226 = call-dynamic "Read AcquisitionD.vi"("error in (no error)"=w3268, "S4ACS_GUI in"=w3267) -> ("error out"=w3224:errorcluster, "Acquisition.lvclass"=w3226:refnum<class "Acquisition.lvclass">, "S4ACS_GUI out"=w3266:refnum<class "S4GUI.lvclass">)  [unwired: 7 in]
          n1227 = call-dynamic "Read enabled.vi"("error in (no error)"=w3224, "Server in"=w3226) -> ("error out"=w3223:errorcluster, "enabled"=w3219:bool, "Server out"=w3225:refnum<class "Acquisition.lvclass">)  [unwired: 7 in]
          n1228 = call "Read connection.vi"("error in (no error)"=w3223, "Server in"=w3225) -> ("error out"=w3255:errorcluster, "connection"=w3239:bool, "Server out"=w3256:refnum<class "Acquisition.lvclass">)  [unwired: 7 in]
          n1229 = And(x=w3239, y=w3219) -> (x .and. y?=w3241:bool)
          n1230 = case shown="True" w3241 {
            tunnel: w3255 -> [w3323 w3343]
            tunnel: [w3323 w3342] -> w3269
            tunnel: w3256 -> [w3324 w3335]
            tunnel: [w3324 w3333] -> w3265
            tunnel: [w3320 u32 0 ("New_State")] -> w3248
            tunnel: w3219 -> [w3319 _]
            frame False {
              n1231 = Select(t=u32 8, s=w3319, f=u32 0) -> (s? t:f=w3320:u32)
            }
            frame True {
              n1232 = call-dynamic "Read Channel.vi"("error in (no error)"=w3343, "Acquisition in"=w3335) -> ("error out"=w3325:errorcluster, "Channel.lvclass"=w3328:refnum<class "Channel.lvclass">, "Acquisition out"=w3334:refnum<class "Acquisition.lvclass">)  [unwired: 7 in]
              n1233 = call-dynamic "Write wait_expose.vi"("error in (no error)"=w3325, "wait_expose"=TRUE, "Channel in"=w3328) -> ("error out"=w3326:errorcluster, "Channel out"=w3327:refnum<class "Channel.lvclass">)  [unwired: 7 in]
              n1234 = call-dynamic "Read State Machine.vi"("error in (no error)"=w3326, "Device in"=w3327) -> ("error out"=w3339:errorcluster, "State Machine.lvclass"=w3341:refnum<class "State Machine.lvclass">, "Device out"=w3337:refnum<class "Channel.lvclass">)  [unwired: 7 in]
              n1235 = call "Next State.vi"("error in (no error)"=w3339, "New_State"=40, "State Machine in"=w3341) -> ("error out"=w3331:errorcluster, "State Machine out"=w3332:refnum<class "State Machine.lvclass">)  [unwired: 7 in]
              n1236 = call-dynamic "Write State Machine.vi"("error in (no error)"=w3331, "State Machine.lvclass"=w3332, "Device in"=w3337) -> ("error out"=w3336:errorcluster, "Device out"=w3338:refnum<class "Channel.lvclass">)  [unwired: 7 in]
              n1237 = call-dynamic "Write Channel.vi"("error in (no error)"=w3336, "Channel.lvclass"=w3338, "Acquisition in"=w3334) -> ("error out"=w3342:errorcluster, "Acquisition out"=w3333:refnum<class "Acquisition.lvclass">)  [unwired: 7 in]
            }
          }
          n1238 = call-dynamic "Write AcquisitionD.vi"("error in (no error)"=w3269, "Acquisition.lvclass"=w3265, "S4ACS_GUI in"=w3266) -> ("error out"=w3264:errorcluster, "S4ACS_GUI out"=w3263:refnum<class "S4GUI.lvclass">)  [unwired: 7 in]
          n1239 = Compound Arithmetic op=ADD(w3251, w3250, w3249, w3248) -> (w3252:u32)
          n1240 = case shown="0, Default" w3252 {
            tunnel: w3247 -> [w3288 _ _ _ _ _ _ _ _ _ _ _ _ _ _ _]
            tunnel: [w3287 u32 1 ("Obs_state") u32 1 ("Obs_state") u32 1 ("Obs_state") u32 1 ("Obs_state") u32 1 ("Obs_state") u32 1 ("Obs_state") u32 1 ("Obs_state") u32 1 ("Obs_state") u32 1 ("Obs_state") u32 1 ("Obs_state") u32 1 ("Obs_state") u32 1 ("Obs_state") u32 1 ("Obs_state") u32 1 ("Obs_state") u32 1 ("Obs_state")] -> w3253
            tunnel: ["" ("Error Msg") "ERROR: Lost channel 1 connection... - HandleObservationSync.vi state 321" ("Error Msg") "ERROR: Lost channel 2 connection...- HandleObservationSync.vi state 321" ("Error Msg") "ERROR: Lost channels 1 and 2 connection...- HandleObservationSync.vi state 321" ("Error Msg") "ERROR: Lost channel 3 connection...- HandleObservationSync.vi state 321" ("Error Msg") "ERROR: Lost channels 1 and  3 connection...- HandleObservationSync.vi state 321" ("Error Msg") "ERROR:  Lost channels 2 and  3 connection...- HandleObservationSync.vi state 321" ("Error Msg") "ERROR:  Lost channels 1, 2 and  3 connection...- HandleObservationSync.vi state 321" ("Error Msg") "ERROR: Lost channel 4 connection...- HandleObservationSync.vi state 321" ("Error Msg") "ERROR:  Lost channels 1 and 4 connection...- HandleObservationSync.vi state 321" ("Error Msg") "ERROR:  Lost channels 2 and 4 connection...- HandleObservationSync.vi state 321" ("Error Msg") "ERROR: Lost channels 1, 2 and 4 connection...- HandleObservationSync.vi state 321" ("Error Msg") "ERROR: Lost channels 3 and 4 connection...- HandleObservationSync.vi state 321" ("Error Msg") "ERROR: Lost channels 1, 3 and 4 connection...- HandleObservationSync.vi state 321" ("Error Msg") "ERROR: Lost channels 2, 3 and 4 connection...- HandleObservationSync.vi state 321" ("Error Msg") "ERROR: Lost channels 1, 2, 3 and 4 connection...- HandleObservationSync.vi state 321" ("Error Msg")] -> w3254
            frame 0, Default {
              n1241 = Increment(x=w3288) -> (x+1=w3287:u32)
            }
            frame 1 {
            }
            frame 2 {
            }
            frame 3 {
            }
            frame 4 {
            }
            frame 5 {
            }
            frame 6 {
            }
            frame 7 {
            }
            frame 8 {
            }
            frame 9 {
            }
            frame 10 {
            }
            frame 11 {
            }
            frame 12 {
            }
            frame 13 {
            }
            frame 14 {
            }
            frame 15 {
            }
          }
          n1242 = Bundle By Name(cluster=w3263, "Obs_state"=w3253, "Error Msg"=w3254) -> (w3280:refnum<class "S4GUI.lvclass">)
        }
        frame 322 {
          # "Espera terminar o envio de WAIT EXPOSE COMMAND para todos os ACS."
          n1243 = call-dynamic "VerifyAcqIdle.vi"("error in (no error)"=w3420, "S4GUI in"=w3419) -> ("error out"=w3425:errorcluster, "idle"=w3424:bool, "S4GUI out"=w3426:refnum<class "S4GUI.lvclass">)  [unwired: 7 in]
          n1244 = disable-structure shown="Enabled" {
            disable-tunnel: w3422 -> [w3429 _]
            disable-tunnel: [w3428 u32 325] -> w3421
            frame Disabled {
              n1245 = Increment(x=w3429) -> (x+1=w3428:u32)
            }
            frame Enabled {
            }
          }
          n1246 = Select(t=w3421, s=w3424, f=w3422) -> (s? t:f=w3423:u32)
          n1247 = Bundle By Name(cluster=w3426, "Obs_state"=w3423) -> (w3427:refnum<class "S4GUI.lvclass">)
        }
        frame 323 {
          n1248 = call-dynamic "Read AcquisitionA.vi"("error in (no error)"=w3493, "S4ACS_GUI in"=w3494) -> ("error out"=w3448:errorcluster, "Acquisition.lvclass"=w3449:refnum<class "Acquisition.lvclass">, "S4ACS_GUI out"=w3496:refnum<class "S4GUI.lvclass">)  [unwired: 7 in]
          n1249 = call-dynamic "Read enabled.vi"("error in (no error)"=w3448, "Server in"=w3449) -> ("error out"=w3447:errorcluster, "enabled"=w3434:bool, "Server out"=w3450:refnum<class "Acquisition.lvclass">)  [unwired: 7 in]
          n1250 = call "Read connection.vi"("error in (no error)"=w3447, "Server in"=w3450) -> ("error out"=w3473:errorcluster, "connection"=w3457:bool, "Server out"=w3474:refnum<class "Acquisition.lvclass">)  [unwired: 7 in]
          n1251 = And(x=w3457, y=w3434) -> (x .and. y?=w3458:bool)
          n1252 = case shown="True" w3458 {
            tunnel: w3474 -> [w3603 w3619]
            tunnel: w3473 -> [w3602 w3618]
            tunnel: [w3603 w3616] -> w3497
            tunnel: [w3602 w3615] -> w3495
            tunnel: [w3599 u32 0 ("New_State")] -> w3463
            tunnel: w3434 -> [w3598 _]
            frame False {
              n1253 = Select(t=u32 1, s=w3598, f=u32 0) -> (s? t:f=w3599:u32)
            }
            frame True {
              n1254 = call-dynamic "Read Channel.vi"("error in (no error)"=w3618, "Acquisition in"=w3619) -> ("error out"=w3611:errorcluster, "Channel.lvclass"=w3610:refnum<class "Channel.lvclass">, "Acquisition out"=w3617:refnum<class "Acquisition.lvclass">)  [unwired: 7 in]
              n1255 = call-dynamic "Read State Machine.vi"("error in (no error)"=w3611, "Device in"=w3610) -> ("error out"=w3612:errorcluster, "State Machine.lvclass"=w3614:refnum<class "State Machine.lvclass">, "Device out"=w3608:refnum<class "Channel.lvclass">)  [unwired: 7 in]
              n1256 = call "Next State.vi"("error in (no error)"=w3612, "New_State"=50, "State Machine in"=w3614) -> ("error out"=w3605:errorcluster, "State Machine out"=w3606:refnum<class "State Machine.lvclass">)  [unwired: 7 in]
              n1257 = call-dynamic "Write State Machine.vi"("error in (no error)"=w3605, "State Machine.lvclass"=w3606, "Device in"=w3608) -> ("error out"=w3607:errorcluster, "Device out"=w3609:refnum<class "Channel.lvclass">)  [unwired: 7 in]
              n1258 = call-dynamic "Write Channel.vi"("error in (no error)"=w3607, "Channel.lvclass"=w3609, "Acquisition in"=w3617) -> ("error out"=w3615:errorcluster, "Acquisition out"=w3616:refnum<class "Acquisition.lvclass">)  [unwired: 7 in]
            }
          }
          n1259 = call-dynamic "Write AcquisitionA.vi"("error in (no error)"=w3495, "Acquisition.lvclass"=w3497, "S4ACS_GUI in"=w3496) -> ("error out"=w3490:errorcluster, "S4ACS_GUI out"=w3491:refnum<class "S4GUI.lvclass">)  [unwired: 7 in]
          n1260 = call "Read AcquisitionB.vi"("error in (no error)"=w3490, "S4ACS_GUI in"=w3491) -> ("error out"=w3444:errorcluster, "Acquisition.lvclass"=w3446:refnum<class "Acquisition.lvclass">, "S4ACS_GUI out"=w3488:refnum<class "S4GUI.lvclass">)  [unwired: 7 in]
          n1261 = call-dynamic "Read enabled.vi"("error in (no error)"=w3444, "Server in"=w3446) -> ("error out"=w3443:errorcluster, "enabled"=w3433:bool, "Server out"=w3445:refnum<class "Acquisition.lvclass">)  [unwired: 7 in]
          n1262 = call "Read connection.vi"("error in (no error)"=w3443, "Server in"=w3445) -> ("error out"=w3471:errorcluster, "connection"=w3455:bool, "Server out"=w3472:refnum<class "Acquisition.lvclass">)  [unwired: 7 in]
          n1263 = And(x=w3455, y=w3433) -> (x .and. y?=w3456:bool)
          n1264 = case shown="True" w3456 {
            tunnel: w3472 -> [w3581 w3597]
            tunnel: w3471 -> [w3580 w3596]
            tunnel: [w3581 w3594] -> w3489
            tunnel: [w3580 w3593] -> w3487
            tunnel: [w3577 u32 0 ("New_State")] -> w3462
            tunnel: w3433 -> [w3576 _]
            frame False {
              n1265 = Select(t=u32 2, s=w3576, f=u32 0) -> (s? t:f=w3577:u32)
            }
            frame True {
              n1266 = call-dynamic "Read Channel.vi"("error in (no error)"=w3596, "Acquisition in"=w3597) -> ("error out"=w3589:errorcluster, "Channel.lvclass"=w3588:refnum<class "Channel.lvclass">, "Acquisition out"=w3595:refnum<class "Acquisition.lvclass">)  [unwired: 7 in]
              n1267 = call-dynamic "Read State Machine.vi"("error in (no error)"=w3589, "Device in"=w3588) -> ("error out"=w3590:errorcluster, "State Machine.lvclass"=w3592:refnum<class "State Machine.lvclass">, "Device out"=w3586:refnum<class "Channel.lvclass">)  [unwired: 7 in]
              n1268 = call "Next State.vi"("error in (no error)"=w3590, "New_State"=50, "State Machine in"=w3592) -> ("error out"=w3583:errorcluster, "State Machine out"=w3584:refnum<class "State Machine.lvclass">)  [unwired: 7 in]
              n1269 = call-dynamic "Write State Machine.vi"("error in (no error)"=w3583, "State Machine.lvclass"=w3584, "Device in"=w3586) -> ("error out"=w3585:errorcluster, "Device out"=w3587:refnum<class "Channel.lvclass">)  [unwired: 7 in]
              n1270 = call-dynamic "Write Channel.vi"("error in (no error)"=w3585, "Channel.lvclass"=w3587, "Acquisition in"=w3595) -> ("error out"=w3593:errorcluster, "Acquisition out"=w3594:refnum<class "Acquisition.lvclass">)  [unwired: 7 in]
